vi "ReadPLC.vi"(7 "PC IP address":string="192.168.1.52", 8 "Error In":errorcluster, 11 "PLCSignals In":T1) -> (0 "Error Out":errorcluster, 3 "PLCSignals Out":T1, 4 "Read errors":string, 6 "Read Error":bool)   [LabVIEW 2018]
uses:
  Clusters/CtrlSignals.ctl
  <vilib>/ethernetip/ethernetip.llb/ethernetip.ctl
  <vilib>/ethernetip/ethernetip.llb/EthernetIP Tag Read DINT.vi
  <vilib>/ethernetip/ethernetip.lvlib
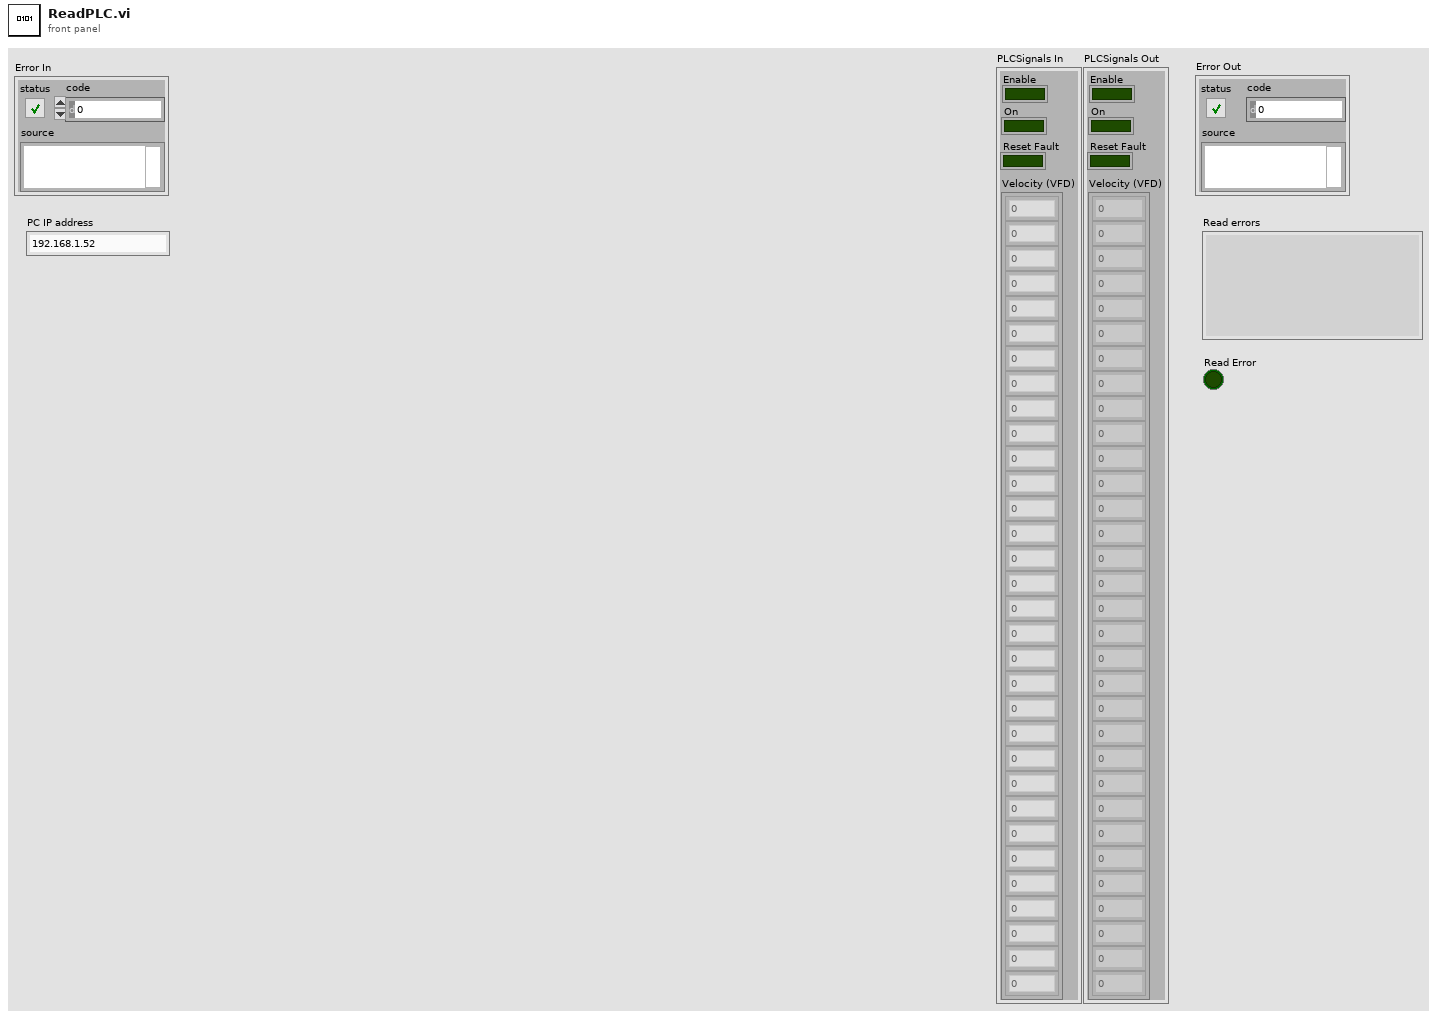
[diagram p1: front panel]
types:
  T1 = typedef "CtrlSignals.ctl" = cluster{"Enable":bool, "On":bool, "Reset Fault":bool, "Velocity (VFD)":i32[]}
  T2 = typedef "ethernetip.lvlib/ethernetip.ctl" = refnum<k21>
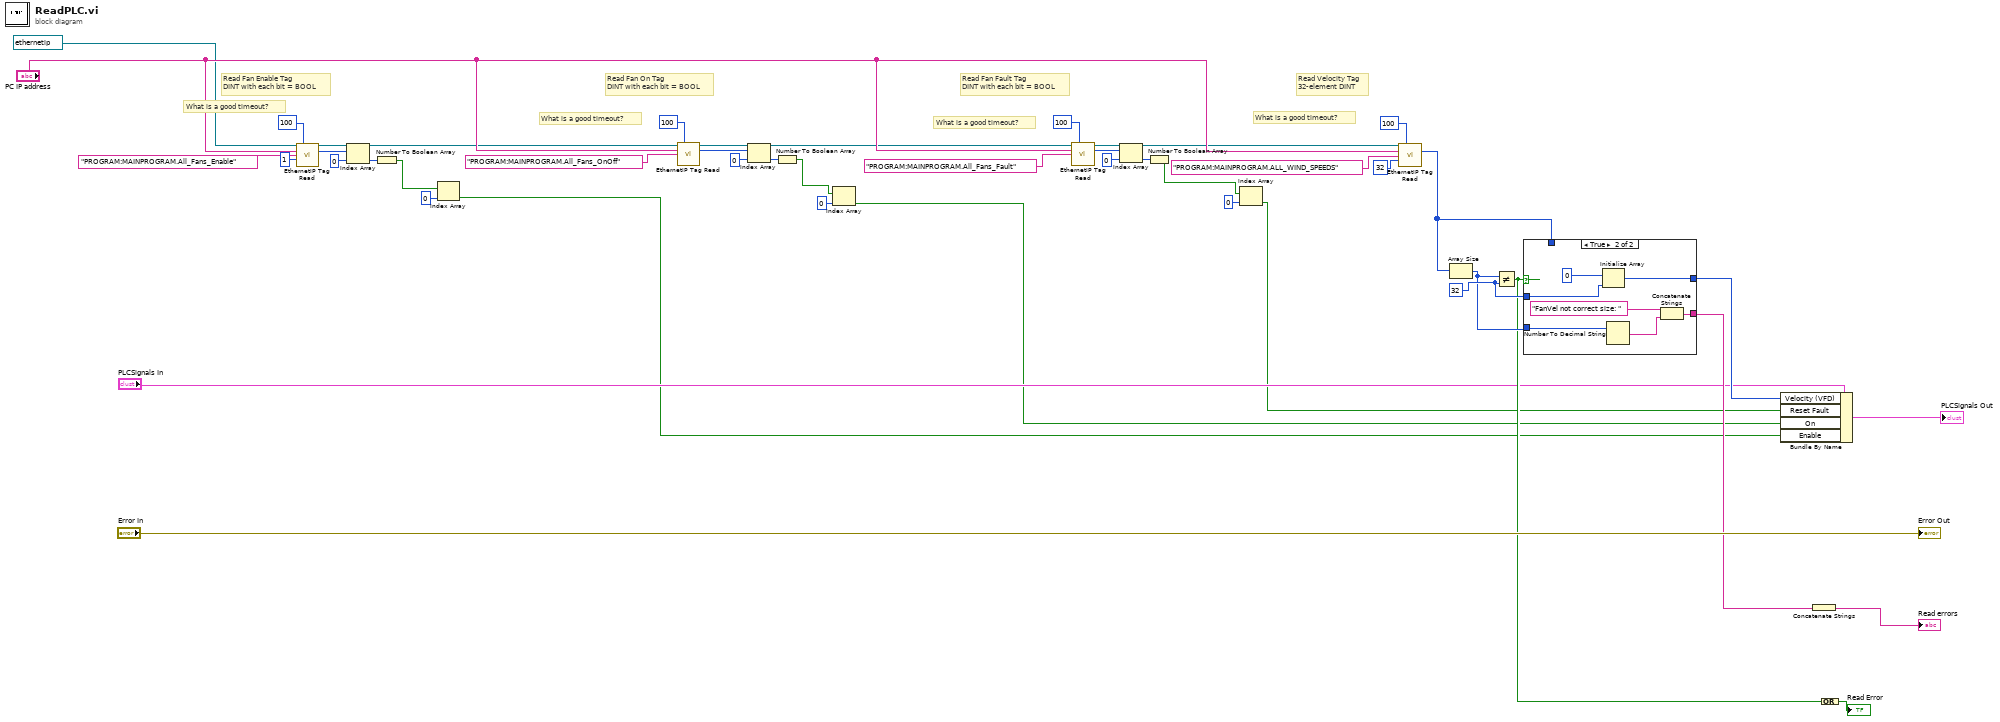
[diagram p0: block diagram]
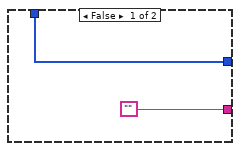
[diagram p2: hidden frame]
diagram:
  w40 = 32 ("y")
  # "What is a good timeout?"
  # "Read Fan Fault Tag\nDINT with each bit = BOOL"
  # "What is a good timeout?"
  # "What is a good timeout?"
  # "Read Fan On Tag\nDINT with each bit = BOOL"
  # "Read Fan Enable Tag\nDINT with each bit = BOOL"
  # "What is a good timeout?"
  # "Read Velocity Tag\n32-element DINT"
  n1 = call-poly <vilib>:"EthernetIP Tag Read.vi"("Session in"=T2 "Default", "Timeout (ms)"=100, "Network Path"="PC IP address", "Tag Name"="PROGRAM:MAINPROGRAM.All_Fans_Enable", "Number of Elements"=u32 1) -> ("Session out"=w16:T2, "Data"=w12:i32[])  [unwired: 8 in, 1 out]
  n2 = Index Array(array=w12, index=0) -> (element=w13:i32)
  n3 = Number To Boolean Array(number=w13) -> (Boolean array=w4:bool[])
  n4 = Index Array(array=w4, index=0) -> (element=w28:bool)
  n5 = call-poly <vilib>:"EthernetIP Tag Read.vi"("Session in"=w16, "Timeout (ms)"=100, "Network Path"="PC IP address", "Tag Name"="PROGRAM:MAINPROGRAM.All_Fans_OnOff") -> ("Session out"=w15:T2, "Data"=w9:i32[])  [unwired: 9 in, 1 out]
  n6 = Index Array(array=w9, index=0) -> (element=w10:i32)
  n7 = Number To Boolean Array(number=w10) -> (Boolean array=w1:bool[])
  n8 = Index Array(array=w1, index=0) -> (element=w27:bool)
  n9 = call-poly <vilib>:"EthernetIP Tag Read.vi"("Session in"=w15, "Timeout (ms)"=100, "Network Path"="PC IP address", "Tag Name"="PROGRAM:MAINPROGRAM.All_Fans_Fault") -> ("Session out"=w34:T2, "Data"=w6:i32[])  [unwired: 9 in, 1 out]
  n10 = Index Array(array=w6, index=0) -> (element=w7:i32)
  n11 = Number To Boolean Array(number=w7) -> (Boolean array=w25:bool[])
  n12 = Index Array(array=w25, index=0) -> (element=w24:bool)
  n13 = call-poly <vilib>:"EthernetIP Tag Read.vi"("Session in"=w34, "Timeout (ms)"=100, "Network Path"="PC IP address", "Tag Name"="PROGRAM:MAINPROGRAM.ALL_WIND_SPEEDS", "Number of Elements"=u32 32) -> ("Data"=w38:i32[])  [unwired: 8 in, 2 out]
  n14 = Array Size(array=w38) -> (size(s)=w39:i32)
  n15 = Not Equal?(x=w39, y=w40) -> (x != y?=w33:bool)
  n16 = case shown="True" w33 {
    tunnel: w40 -> [_ w53]
    tunnel: [w45 w52] -> w36
    tunnel: ["" w50] -> w37
    tunnel: w39 -> [_ w48]
    tunnel: w38 -> [w45 _]
    frame False {
    }
    frame True {
      n17 = Initialize Array(0, w53) -> (w52:i32[])
      n18 = Number To Decimal String(number=w48) -> (decimal integer string=w49:string)  [unwired: 1 in]
      n19 = Concatenate Strings("FanVel not correct size: ", w49) -> (w50:string)
    }
  }
  n20 = Bundle By Name(cluster="PLCSignals In", "Velocity (VFD)"=w36, "Reset Fault"=w24, "On"=w27, "Enable"=w28) -> (→"PLCSignals Out":T1)
  n21 = Concatenate Strings(w37) -> (→"Read errors":string)
  n22 = Compound Arithmetic op=OR(w33) -> (→"Read Error":bool)
  "Error Out" <- "Error In"
